vi "Test.vi"() -> ()   [LabVIEW 2022 SP3]
panel:
  out "OutCluster":T1
  out "ErrorOut":errorcluster
  in  "stop":bool
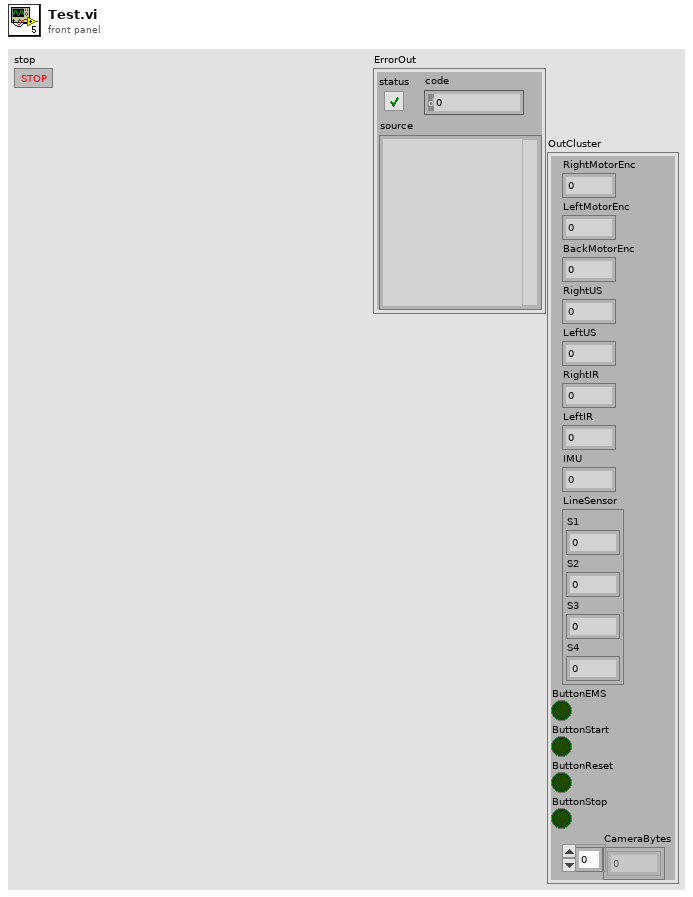
[diagram p1: front panel]
types:
  T1 = cluster{"RightMotorEnc":dbl, "LeftMotorEnc":dbl, "BackMotorEnc":dbl, "RightUS":dbl, "LeftUS":dbl, "RightIR":dbl, "LeftIR":dbl, "IMU":dbl, "LineSensor":cluster{"S1":dbl, "S2":dbl, "S3":dbl, "S4":dbl}, "ButtonEMS":bool, "ButtonStart":bool, "ButtonReset":bool, "ButtonStop":bool, "CameraBytes":u8[]}
  T2 = cluster{"RightMotorSpeed":dbl, "LeftMotorSpeed":dbl, "BackMotorSpeed":dbl, "ResetRightEnc":bool, "ResetLeftEnc":bool, "ResetBackEnc":bool, "ResetIMU":bool, "LedGreen":bool, "LedRed":bool}
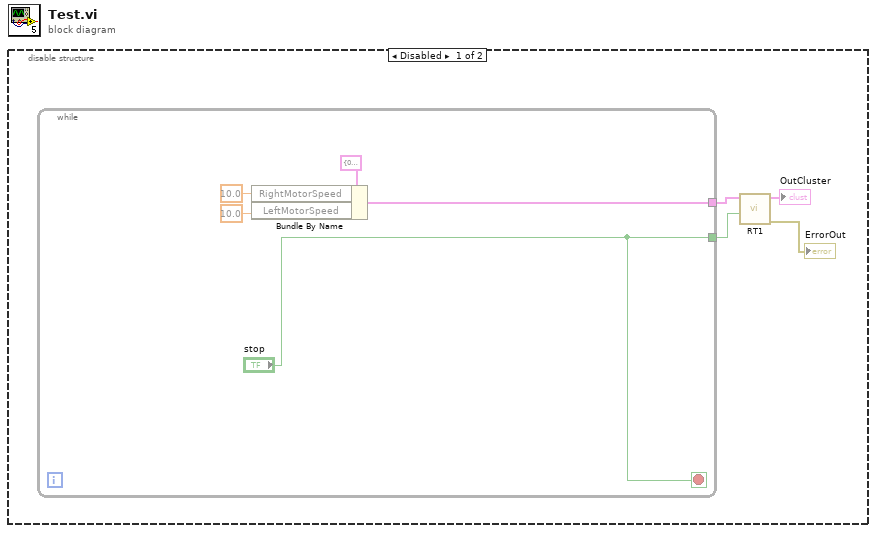
[diagram p0: block diagram]
diagram:
  n1 = disable-structure shown="Disabled" {
    frame Disabled {
      n2 = while {
        tunnel: ["stop"] -> w2
        tunnel: [w6] -> w3
        stop <- "stop" stop-if-true
        n3 = Bundle By Name(cluster=T2 {"RightMotorSpeed"=0.0, "LeftMotorSpeed"=0.0, "BackMotorSpeed"=0.0, "ResetRightEnc"=FALSE, "ResetLeftEnc"=FALSE, "ResetBackEnc"=FALSE, "ResetIMU"=FALSE, "LedGreen"=FALSE, "LedRed"=FALSE} ("InCluster"), "RightMotorSpeed"=10.0, "LeftMotorSpeed"=10.0) -> (w6:T2)
      }
      n4 = call "RT1.vi"("Disconnect"=w2, "InCluster"=w3) -> ("ErrorOut"=→"ErrorOut":errorcluster, "OutCluster"=→"OutCluster":T1)  [unwired: 7 in, 1 out]
    }
    frame Enabled {
    }
  }
